vi "Scan.vi"(11 "IScanner In":refnum<class "IScanner.lvclass">) -> (3 "IScanner Out":refnum<class "IScanner.lvclass">)   [LabVIEW 2018, in "IScanner.lvclass"]
uses:
  IScanner.lvclass
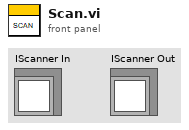
[diagram p1: front panel]
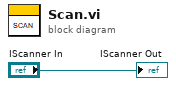
[diagram p0: block diagram]
diagram:
  "IScanner Out" <- "IScanner In"
